vi "计算器.vi"() -> ()   [LabVIEW 2018]
panel:
  out "除":bool
  in  "乘":bool
  in  "减":bool
  in  "加":bool
  out "结果":dbl format="%#_3g"
  in  "输入 2":dbl
  in  "输入1":dbl
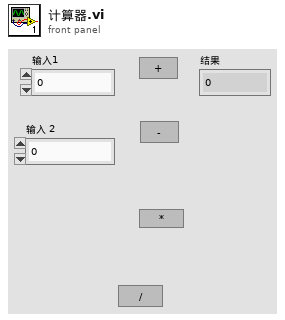
[diagram p1: front panel]
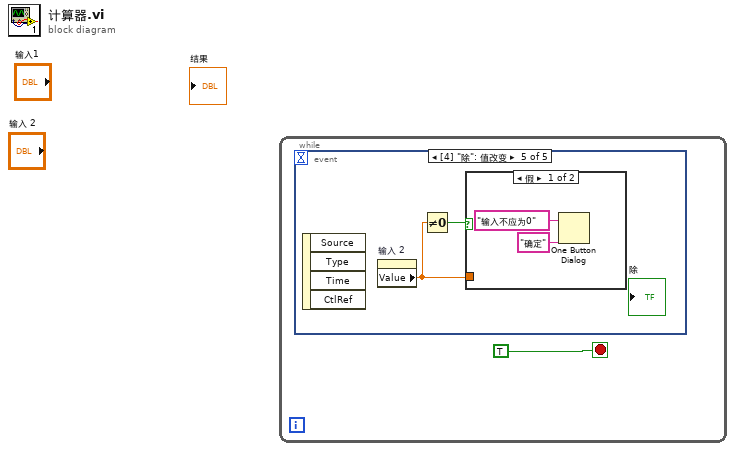
[diagram p0: block diagram]
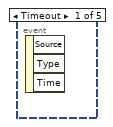
[diagram p2: hidden frame]
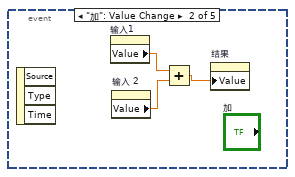
[diagram p3: hidden frame]
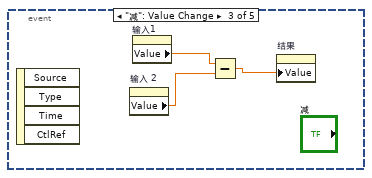
[diagram p4: hidden frame]
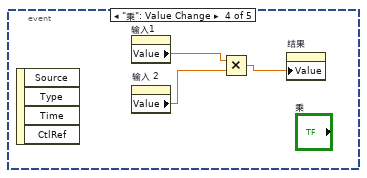
[diagram p5: hidden frame]
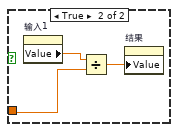
[diagram p6: hidden frame]
diagram:
  n1 = while {
    stop <- TRUE stop-if-true
    n2 = event shown="[4] \"除\": 值改变" {
      selector: _ -> [_ _ _ _ _]
      dyn-events: _ -> [_ _ _ _ _]
      timeout: _ -> [_ _ _ _ _]
      event Timeout {
        n3 = event-data() -> ()  [unwired: 1 in, 3 out]
      }
      event "加": Value Change {
        n4 = event-data() -> ()  [unwired: 1 in, 3 out]
        n5 = property on="输入1" class="DigNum (严格)"() -> ("Value"=w4:dbl)  [unwired: 2 in, 2 out]
        n6 = property on="输入 2" class="DigNum (严格)"() -> ("Value"=w3:dbl)  [unwired: 2 in, 2 out]
        n7 = Add(x=w4, y=w3) -> (x+y=w2:dbl)
        n8 = property on="结果" class="DigNum (严格)"("Value"=w2) -> ()  [unwired: 2 in, 2 out]
      }
      event "减": Value Change {
        n9 = event-data() -> ()  [unwired: 1 in, 4 out]
        n10 = property on="输入 2" class="DigNum (严格)"() -> ("Value"=w5:dbl)  [unwired: 2 in, 2 out]
        n11 = property on="输入1" class="DigNum (严格)"() -> ("Value"=w6:dbl)  [unwired: 2 in, 2 out]
        n12 = Subtract(x=w6, y=w5) -> (x-y=w7:dbl)
        n13 = property on="结果" class="DigNum (严格)"("Value"=w7) -> ()  [unwired: 2 in, 2 out]
      }
      event "乘": Value Change {
        n14 = event-data() -> ()  [unwired: 1 in, 4 out]
        n15 = property on="输入1" class="DigNum (严格)"() -> ("Value"=w9:dbl)  [unwired: 2 in, 2 out]
        n16 = property on="输入 2" class="DigNum (严格)"() -> ("Value"=w8:dbl)  [unwired: 2 in, 2 out]
        n17 = Multiply(x=w9, y=w8) -> (x*y=w10:dbl)
        n18 = property on="结果" class="DigNum (严格)"("Value"=w10) -> ()  [unwired: 2 in, 2 out]
      }
      event "除": Value Change {
        n19 = event-data() -> ()  [unwired: 1 in, 4 out]
        n20 = property on="输入 2" class="DigNum (严格)"() -> ("Value"=w12:dbl)  [unwired: 2 in, 2 out]
        n21 = Not Equal To 0?(x=w12) -> (x != 0?=w11:bool)
        n22 = case shown="假" w11 {
          tunnel: w12 -> [_ w16]
          frame False {
            n23 = One Button Dialog(message="输入不应为0" ("消息"), button name ("OK")="确定" ("按钮名称（“确定”）")) -> ()  [unwired: 1 out]
          }
          frame True {
            n24 = property on="输入1" class="DigNum (严格)"() -> ("Value"=w15:dbl)  [unwired: 2 in, 2 out]
            n25 = Divide(x=w15, y=w16) -> (x/y=w17:dbl)
            n26 = property on="结果" class="DigNum (严格)"("Value"=w17) -> ()  [unwired: 2 in, 2 out]
          }
        }
      }
    }
  }
